vi "UpdateLotTable.vi"(8 "error in (no error)":errorcluster, 11 "LotData in":refnum<class "LotData.lvclass">) -> (0 "error out":errorcluster, 3 "LotData out":refnum<class "LotData.lvclass">)   [LabVIEW 2012, in "LotData.lvclass"]
uses:
  LotData.lvclass
  LotData.lvclass/LotData.ctl
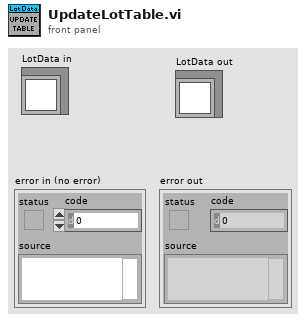
[diagram p1: front panel]
types:
  T1 = typedef "TestData.ctl" = cluster{"20mA Data":cluster{"Area":string, "Current,mA":dbl, "Power":dbl, "WL":dbl, "Voltage":dbl, "Knee Current":dbl, "Reverse":dbl}, "50mA Data":cluster{"Area":string, "Current,mA":dbl, "Power":dbl, "WL":dbl, "Voltage":dbl}}
  T2 = cluster{"Area":string, "Current,mA":dbl, "Power":dbl, "WL":dbl, "Voltage":dbl, "Knee Current":dbl, "Reverse":dbl}
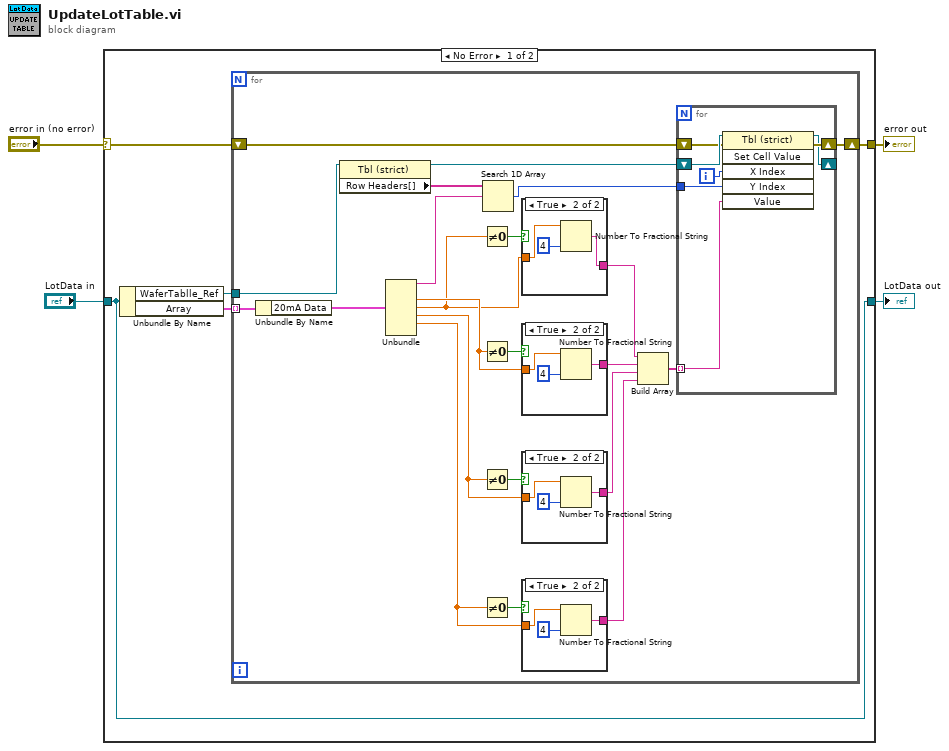
[diagram p0: block diagram]
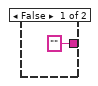
[diagram p2: hidden frame]
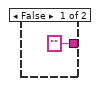
[diagram p3: hidden frame]
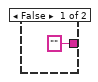
[diagram p4: hidden frame]
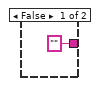
[diagram p5: hidden frame]
diagram:
  n1 = case shown="No Error" "error in (no error)" {
    selector: "error in (no error)" -> [w6 w56]
    tunnel: [w7 w56] -> w3
    tunnel: [w5 w55] -> w1
    tunnel: "LotData in" -> [w5 w55]
    frame No Error {
      n2 = Unbundle By Name(w5) -> ("WaferTablle_Ref"=w8:refnum<vi>, "Array"=w9:T1[])
      n3 = for {
        tunnel: w9 -> [w28] mode=indexing
        tunnel: w8 -> [w27]
        shift-right: [w23] -> w7
        shift-left: w6 -> [w22]
        n4 = Unbundle By Name(w28) -> ("20mA Data"=w31:T2)
        n5 = property class="Tbl (strict)"(reference=w27) -> (reference out=w26:refnum<vi>, "Row Headers[]"=w30:string[])  [unwired: 1 in, 1 out]
        n6 = Unbundle(w31) -> ("Area"=w29:string, "Power"=w20:dbl, "WL"=w14:dbl, "Voltage"=w15:dbl, "Knee Current"=w16:dbl)  [unwired: 2 out]
        n7 = Not Equal To 0?(x=w14) -> (x != 0?=w19:bool)
        n8 = Not Equal To 0?(x=w20) -> (x != 0?=w21:bool)
        n9 = Not Equal To 0?(x=w15) -> (x != 0?=w18:bool)
        n10 = Not Equal To 0?(x=w16) -> (x != 0?=w17:bool)
        n11 = Search 1D Array(1D array=w30, element=w29) -> (index of element=w25:i32)  [unwired: 1 in]
        n12 = case shown="True" w19 {
          tunnel: ["" ("F-format string") w42] -> w12
          tunnel: w14 -> [_ w41]
          frame False {
          }
          frame True {
            n13 = Number To Fractional String(number=w41, precision (6)=i16 4) -> (F-format string=w42:string)  [unwired: 2 in]
          }
        }
        n14 = case shown="True" w21 {
          tunnel: w20 -> [_ w47]
          tunnel: ["" ("F-format string") w45] -> w13
          frame False {
          }
          frame True {
            n15 = Number To Fractional String(number=w47, precision (6)=i16 4) -> (F-format string=w45:string)  [unwired: 2 in]
          }
        }
        n16 = case shown="True" w18 {
          tunnel: ["" ("F-format string") w38] -> w11
          tunnel: w15 -> [_ w37]
          frame False {
          }
          frame True {
            n17 = Number To Fractional String(number=w37, precision (6)=i16 4) -> (F-format string=w38:string)  [unwired: 2 in]
          }
        }
        n18 = case shown="True" w17 {
          tunnel: ["" ("F-format string") w34] -> w10
          tunnel: w16 -> [_ w33]
          frame False {
          }
          frame True {
            n19 = Number To Fractional String(number=w33, precision (6)=i16 4) -> (F-format string=w34:string)  [unwired: 2 in]
          }
        }
        n20 = Build Array(w12, w13, w11, w10) -> (w24:string[])
        n21 = for {
          tunnel: w24 -> [w51] mode=indexing
          tunnel: w25 -> [w53]
          shift-right: [w49] -> w23
          shift-left: w22 -> [w50]
          shift-right: [w48] -> _
          shift-left: w26 -> [w54]
          i -> [w52]
          n22 = invoke class="Tbl (strict)" method="Set Cell Value"(reference=w54, error in=w50, "X Index"=w52, "Y Index"=w53, "Value"=w51) -> (reference out=w48:refnum<vi>, error out=w49:errorcluster)  [unwired: 1 in, 4 out]
        }
      }
    }
    frame Error {
    }
  }
  "error out" <- w3
  "LotData out" <- w1
